vi "SeCrTs-Sequence separator.vi"(5 "Sequence Folder Path":path, 11 "error  in":errorcluster) -> (4 "AI":T1(array[cluster]), 6 "AO":T1(array[cluster]), 8 "DI":T1(array[cluster]), 10 "DO":T1(array[cluster]), 15 "error out":errorcluster)   [LabVIEW 2022 SP3]
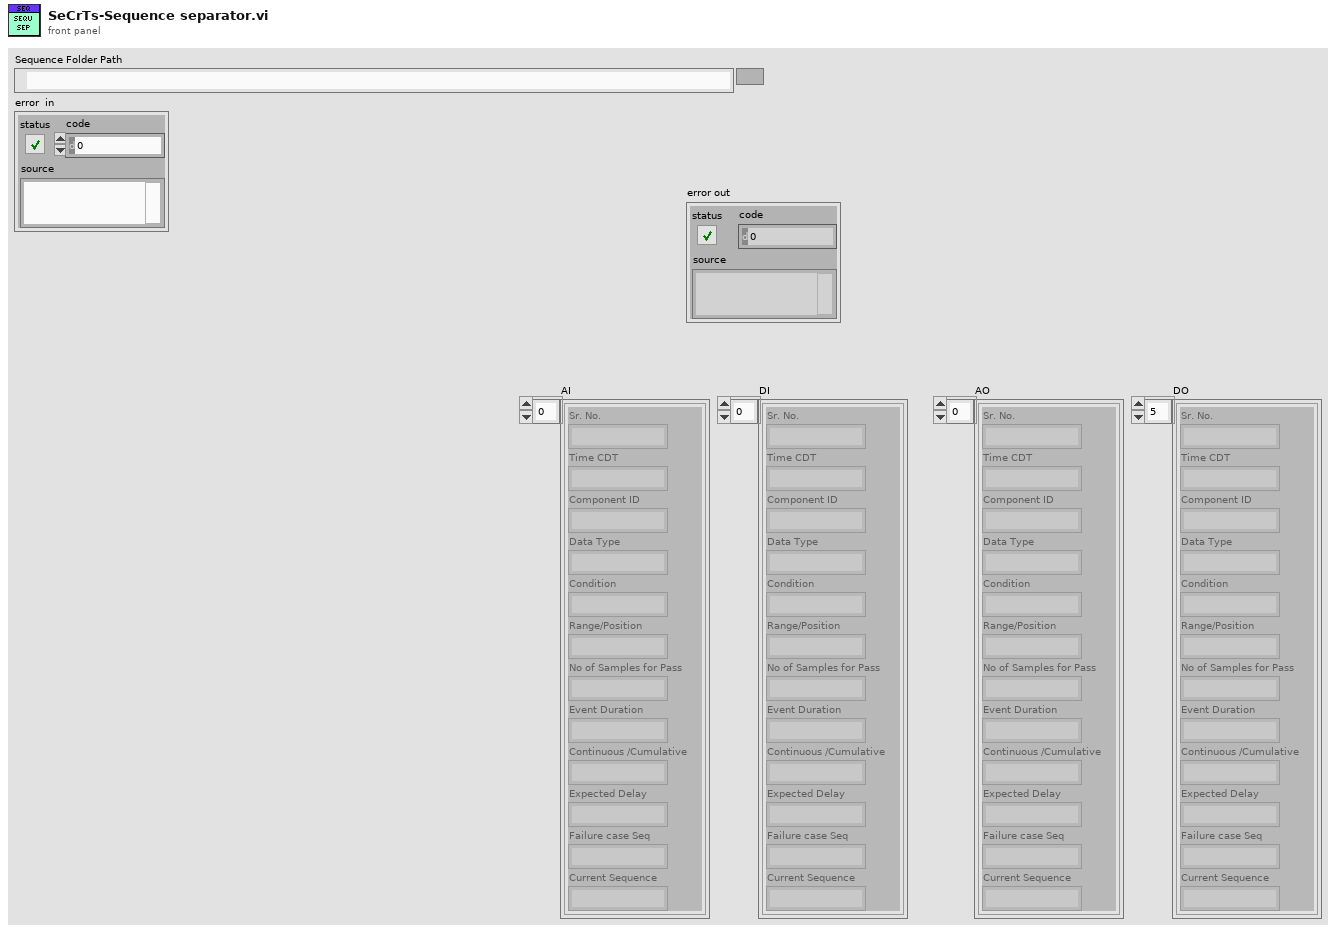
[diagram p1: front panel]
types:
  T1 = cluster{"Sr. No.":string, "Time CDT":string, "Component ID":string, "Data Type":string, "Condition":string, "Range/Position":string, "No of Samples for Pass":string, "Event Duration":string, "Continuous /Cumulative":string, "Expected Delay":string, "Failure case Seq":string, "Current Sequence":string}[]
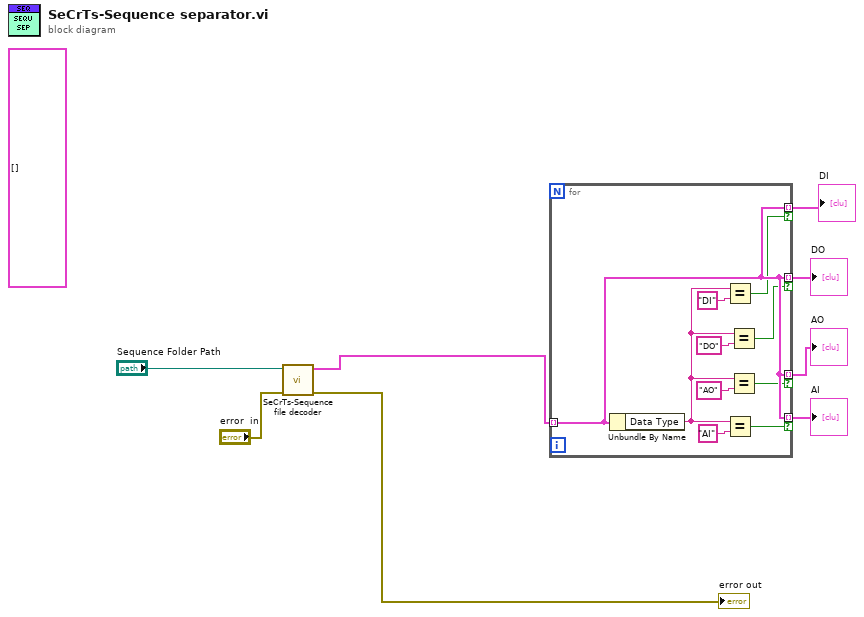
[diagram p0: block diagram]
diagram:
  (unwired) T1 [] ("Seq in")
  n1 = call "SeCrTs-Sequence file decoder.vi"("error in (no error)"="error  in", "file path (dialog if empty)"="Sequence Folder Path") -> ("error out"=→"error out":errorcluster, "Seq in"=w2:T1)  [unwired: 8 in]
  n2 = for {
    tunnel: w2 -> [w12] mode=indexing
    tunnel: [w12] -> w5 mode=indexing if=w17
    tunnel: [w12] -> w4 mode=indexing if=w11
    tunnel: [w12] -> w1 mode=indexing if=w10
    tunnel: [w12] -> w3 mode=indexing if=w9
    n3 = Unbundle By Name(w12) -> ("Data Type"=w13:string)
    n4 = Equal?(x=w13, y="DI") -> (x = y?=w10:bool)
    n5 = Equal?(x=w13, y="AI") -> (x = y?=w17:bool)
    n6 = Equal?(x=w13, y="DO") -> (x = y?=w9:bool)
    n7 = Equal?(x=w13, y="AO") -> (x = y?=w11:bool)
  }
  "AI" <- w5
  "AO" <- w4
  "DI" <- w1
  "DO" <- w3
